vi "Read Block Data (SubVI).vi"(11 "Array In":u64[](array[numeric])) -> (3 "Array Out":u8[][](array[numeric]))   [LabVIEW 2015]
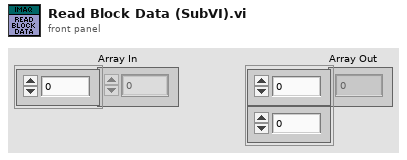
[diagram p1: front panel]
types:
  T1 = enum16{"big-endian, network order", "native, host order", "little-endian"}
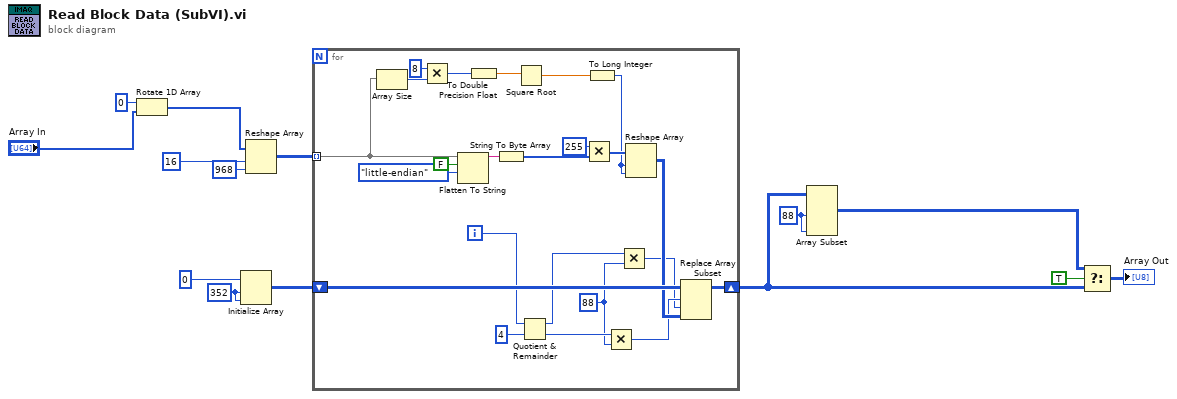
[diagram p0: block diagram]
diagram:
  w12 = 88 ("length")
  w9 = 352 ("dimension size")
  n1 = Rotate 1D Array(1:"Array In", 2:0 ("n")) -> (0:w2:u64[])
  n2 = Initialize Array(u8 0 ("element"), w9, w9) -> (w10:u8[][])
  n3 = Reshape Array(w2, 16 ("dimension size"), 968 ("dimension size")) -> (w6:u64[][])
  n4 = for {
    tunnel: w6 -> [w25] mode=indexing
    shift-right: [w23] -> w11
    shift-left: w10 -> [w24]
    i -> [w21]
    w18 = 88 ("y")
    n5 = Array Size(array=w25) -> (size(s)=w32:i32)
    n6 = Multiply(x=8, y=w32) -> (x*y=w30:i32)
    n7 = Flatten To String(anything=w25, prepend array or string size? (T)=FALSE, byte order (0:big-endian, network order)=T1."little-endian") -> (data string=w36:string)  [unwired: 1 in, 2 out]
    n8 = To Double Precision Float(number=w30) -> (double precision float=w29:dbl)
    n9 = String To Byte Array(string=w36) -> (unsigned byte array=w35:u8[])
    n10 = Square Root(x=w29) -> (sqrt(x)=w28:dbl)
    n11 = Quotient & Remainder(x=w21, y=4) -> (x-y*floor(x/y)=w17:i32, floor(x/y)=w19:i32)
    n12 = Multiply(x=u8 255 ("dimension size"), y=w35) -> (x*y=w34:u8[])
    n13 = To Long Integer(number=w28) -> (32bit integer=w27:i32)
    n14 = Multiply(x=w19, y=w18) -> (x*y=w16:i32)
    n15 = Multiply(x=w17, y=w18) -> (x*y=w15:i32)
    n16 = Reshape Array(w34, w27, w27) -> (w22:u8[][])
    n17 = Replace Array Subset(array=w24, new element=w22, index (row)=w16, index (col)=w15) -> (w23:u8[][])
  }
  n18 = Array Subset(array=w11, length (row)=w12, length (col)=w12) -> (w1:u8[][])  [unwired: 2 in]
  n19 = Select(t=w1, s=TRUE, f=w11) -> (s? t:f=→"Array Out":u8[][])
